vi "总磷氨氮测量数据储存.vi"   [LabVIEW 2016, in "斯坦道仪器.lvlib"]
types:
  T1 = cluster{"时间标识":timestamp, "监测值":sgl, "单位":u16, "数据标识":string, "因子编码":u32, "标样参考值":sgl, "F0":sgl, "F1":sgl, "F2":sgl, "F3":sgl, "F4":sgl, "F5":sgl, "F6":sgl, "F7":sgl, "X":sgl, "温度":sgl, "湿度":sgl, "量程标识":string}
  T2 = enum16{"维护数据", "水样测试", "标样核查", "零点核查", "跨度核查", "空白测试", "平行样测试", "加标回收", "空白校准", "标样校准", "初始化（清洗）"}
  T3 = cluster{"系统时间":timestamp, "工作状态":enum16{"空闲", "水样测试", "标样核查", "零点核查", "跨度核查", "空白测试", "平行样测试", "加标回收", "空白校准", "标样校准", "初始化（清洗）"}, "测量模式":enum16{"待机", "连续模式", "周期模式", "定点模式", "受控模式", "手动模式"}, "告警代码":enum16{"无告警", "缺试剂告警", "缺水样告警", "缺蒸馏水告警", "缺标液告警", "仪表漏液告警", "标定异常告警", "超量程告警", "加热异常", "低试剂预警", "超上限告警", "超下限告警", "仪表内部其他异常", "滴定异常告警", "电极异常告警", "量程切换告警", "参数设置告警", "PH电极电位异常", "电导率电极异常", "浊度光度异常", "溶解氧电极异常", "溶解氧光强异常", "温度异常告警", "PH异常告警", "溶解氧异常告警", "电导率异常告警", "浊度异常告警", "叶绿素异常告警", "藻密度异常告警", "蓝绿藻异常告警", "ORP异常告警", "氨氮异常告警", "清洁刷异常告警", "SD卡异常告警", "蓝牙异常告警", "Wifi异常告警", "流程异常告警"}, "故障代码":enum16{"无故障", "电机故障", "温度故障", "通讯故障", "滴定故障"}, "日志代码":u16, "软件版本":u16, "F0":sgl, "F1":sgl, "F2":sgl, "F3":sgl, "T":sgl, "H":sgl, "id":u16, "flowid":u16, "量程":u16}
  T4 = enum16{"空闲", "水样测试", "标样核查", "零点核查", "跨度核查", "空白测试", "平行样测试", "加标回收", "空白校准", "标样校准", "初始化（清洗）"}
  T5 = cluster{"因子编码":u32, "单位":u16, "标样参考值":sgl, "水样数据时间":timestamp, "水样实测值":sgl, "水样数据标识":string, "标样数据时间":timestamp, "标样实测值":sgl, "标样数据标识":string, "空白数据时间":timestamp, "空白实测值":sgl, "空白数据标识":string, "零点核查数据时间":timestamp, "零点核查实测值":sgl, "零点核查数据标识":string, "跨度核查数据时间":timestamp, "跨度核查实测值":sgl, "跨度核查数据标识":string, "加标回收数据时间":timestamp, "加标回收实测值":sgl, "加标回收数据标识":string, "平行样数据时间":timestamp, "平行样实测值":sgl, "平行样数据标识":string, "F0":sgl, "F1":sgl, "F2":sgl, "F3":sgl, "F4":sgl, "F5":sgl, "F6":sgl, "F7":sgl, "温度":sgl, "湿度":sgl, "X值":sgl}
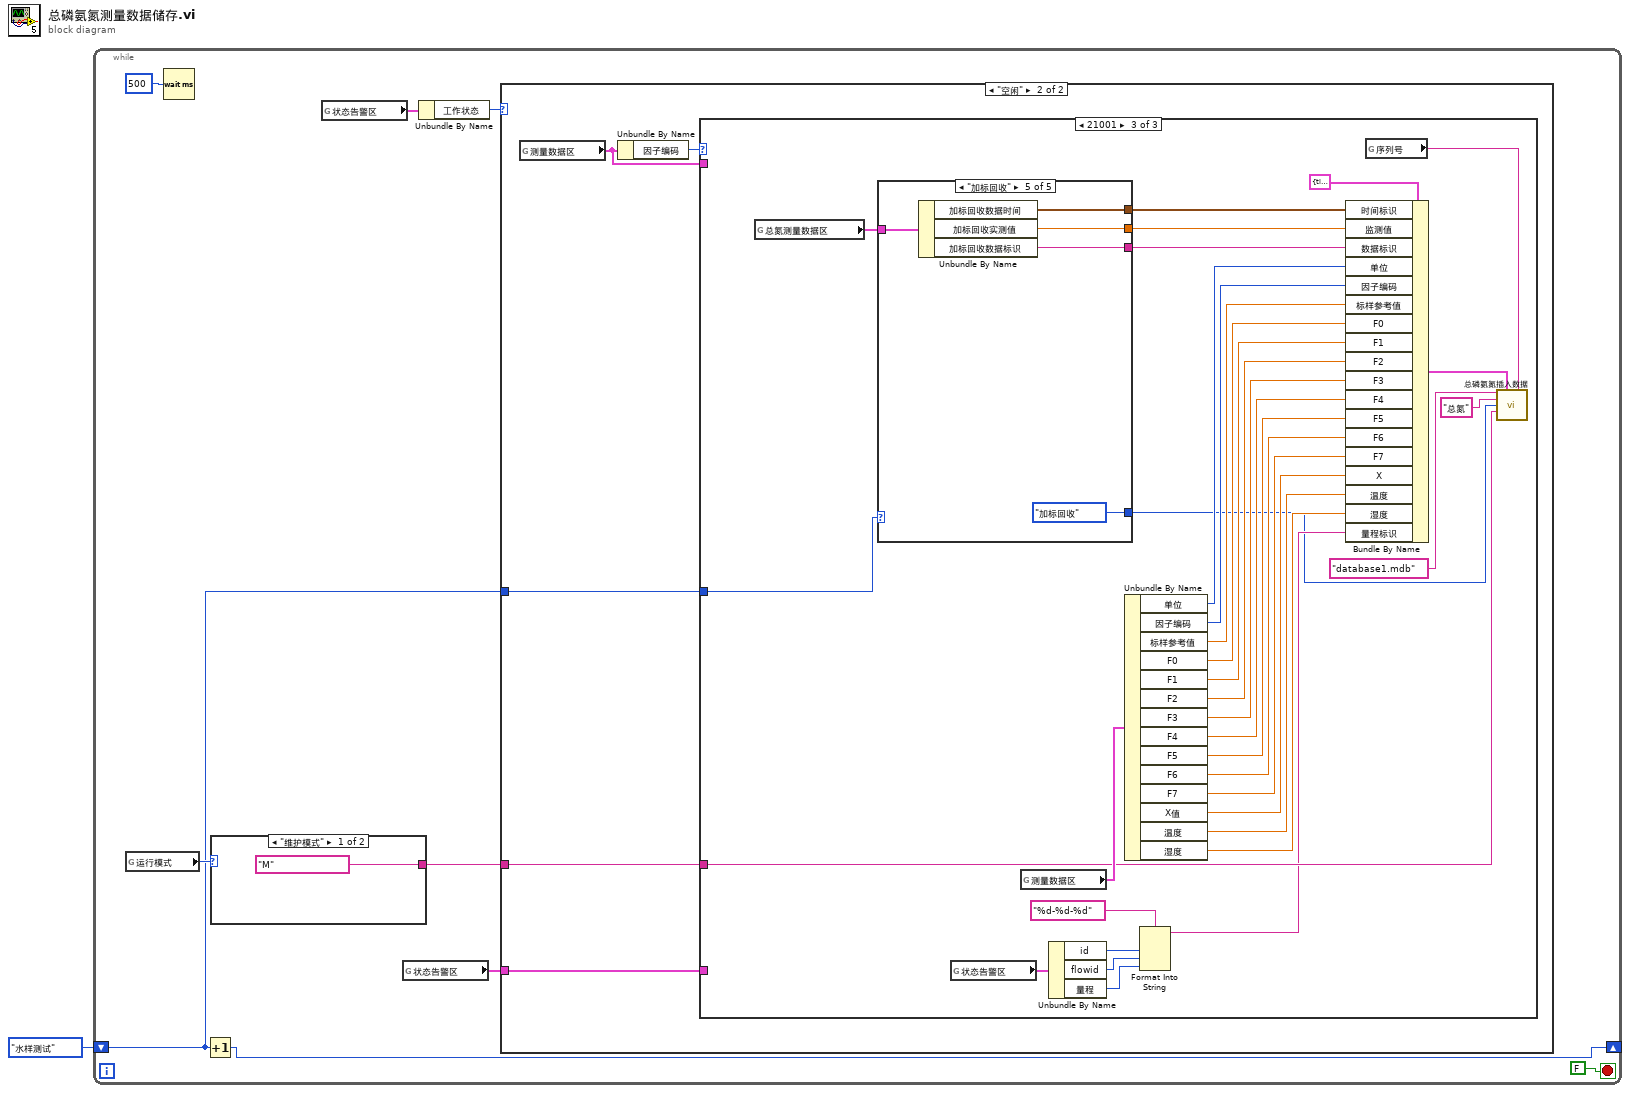
[diagram p0: block diagram]
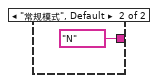
[diagram p2: hidden frame]
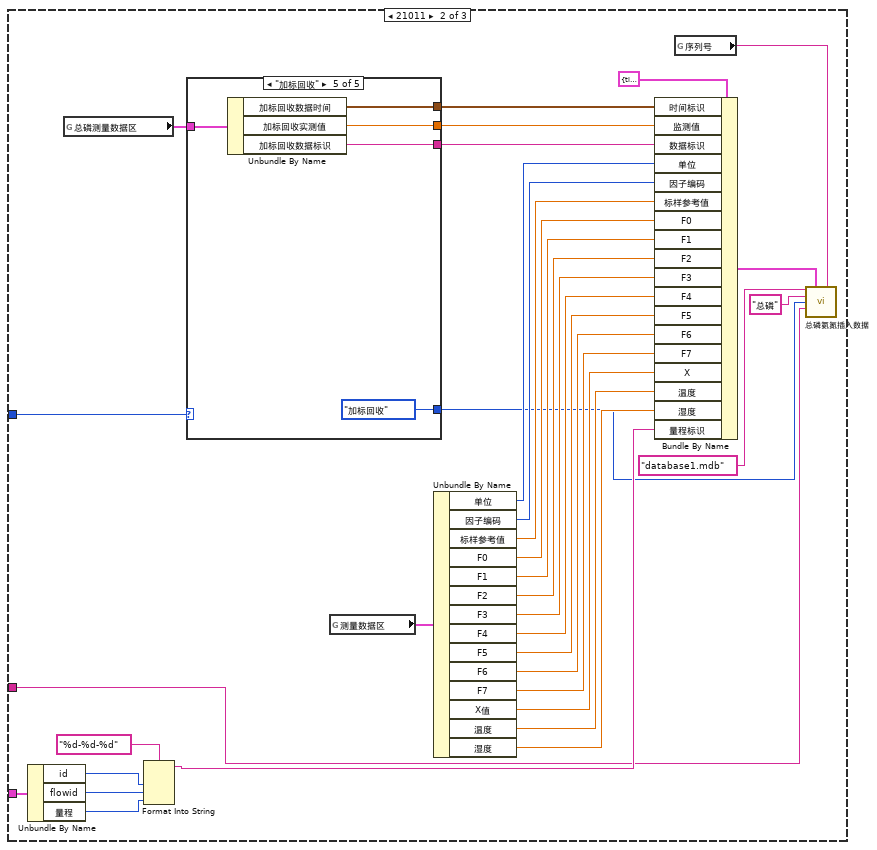
[diagram p5: hidden frame]
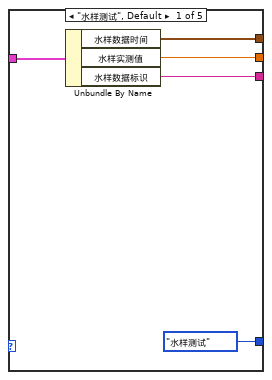
[diagram p6: hidden frame]
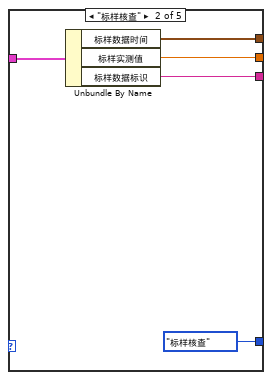
[diagram p7: hidden frame]
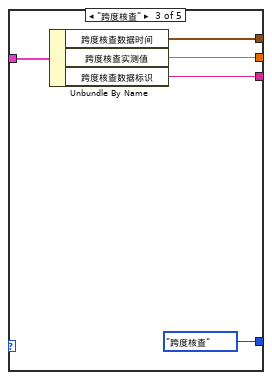
[diagram p8: hidden frame]
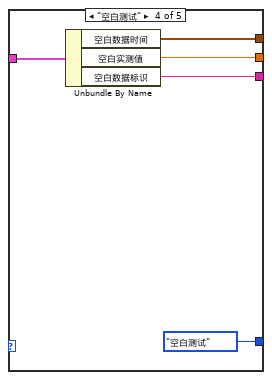
[diagram p9: hidden frame]
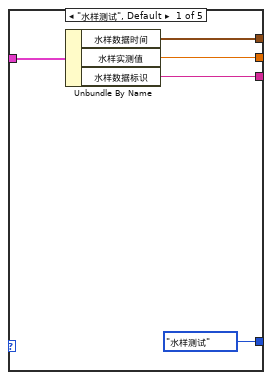
[diagram p10: hidden frame]
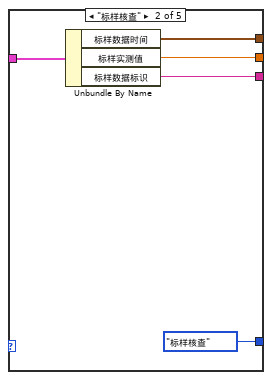
[diagram p11: hidden frame]
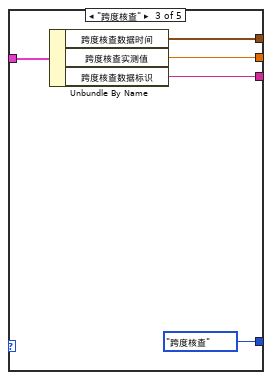
[diagram p12: hidden frame]
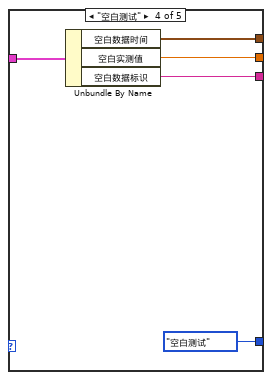
[diagram p13: hidden frame]
diagram:
  n1 = while {
    shift-right: [w4] -> _
    shift-left: enum16{"水样测试", "标样核查", "跨度核查", "空白测试", "加标回收"}."水样测试" ("测量模式") -> [w3]
    stop <- FALSE stop-if-true
    n2 = global read "系统变量.vi" "运行模式"() -> (w6:enum16{"维护模式", "常规模式", "应急模式", "质控模式"})
    n3 = Wait (ms)(milliseconds to wait=u32 500 ("等待时间（毫秒）")) -> ()  [unwired: 1 out]
    n4 = Increment(x=w3) -> (x+1=w4:enum16{"水样测试", "标样核查", "跨度核查", "空白测试", "加标回收"})
    n5 = case shown="\"维护模式\"" w6 {
      tunnel: ["M" ("数据标记表") "N" ("数据标记表")] -> w5
      frame "维护模式" {
      }
      frame "常规模式", Default {
      }
    }
    n6 = global read "VAR总磷氨氮全局变量.vi" "状态告警区"() -> (w8:T3)
    n7 = global read "VAR总磷氨氮全局变量.vi" "状态告警区"() -> (w2:T3)
    n8 = Unbundle By Name(w8) -> ("工作状态"=w7:T4)
    n9 = case shown="\"空闲\"" w7 {
      tunnel: w5 -> [_ w15]
      tunnel: w3 -> [_ w14]
      tunnel: w2 -> [_ w13]
      frame Default {
      }
      frame "空闲" {
        n10 = global read "VAR总磷氨氮全局变量.vi" "测量数据区"() -> (w17:T5)
        n11 = Unbundle By Name(w17) -> ("因子编码"=w16:u32)
        n12 = case shown="21001" w16 {
          tunnel: w17 -> [_ _ _]
          tunnel: w15 -> [_ w20 w96]
          tunnel: w14 -> [_ w19 w81]
          tunnel: w13 -> [_ w18 _]
          frame Default {
          }
          frame 21011 {
            n13 = Unbundle By Name(w18) -> ("id"=w50:u16, "flowid"=w33:u16, "量程"=w32:u16)
            n14 = global read "VAR总磷氨氮全局变量.vi" "总磷测量数据区"() -> (w49:T5)
            n15 = Format Into String(format string="%d-%d-%d" ("格式字符串"), w50, w33, w32) -> (resulting string=w34:string)  [unwired: 2 in, 1 out]
            n16 = case shown="\"加标回收\"" w19 {
              tunnel: w49 -> [w55 w60 w65 w70 w75]
              tunnel: [w54 w59 w64 w69 w74] -> w24
              tunnel: [w53 w58 w63 w68 w73] -> w25
              tunnel: [w52 w57 w62 w67 w72] -> w26
              tunnel: [T2."水样测试" ("测量模式") T2."标样核查" ("测量模式") T2."跨度核查" ("测量模式") T2."空白测试" ("测量模式") T2."加标回收" ("测量模式")] -> w23
              frame "水样测试", Default {
                n17 = Unbundle By Name(w55) -> ("水样数据时间"=w54:timestamp, "水样实测值"=w53:sgl, "水样数据标识"=w52:string)
              }
              frame "标样核查" {
                n18 = Unbundle By Name(w60) -> ("标样数据时间"=w59:timestamp, "标样实测值"=w58:sgl, "标样数据标识"=w57:string)
              }
              frame "跨度核查" {
                n19 = Unbundle By Name(w65) -> ("跨度核查数据时间"=w64:timestamp, "跨度核查实测值"=w63:sgl, "跨度核查数据标识"=w62:string)
              }
              frame "空白测试" {
                n20 = Unbundle By Name(w70) -> ("空白数据时间"=w69:timestamp, "空白实测值"=w68:sgl, "空白数据标识"=w67:string)
              }
              frame "加标回收" {
                n21 = Unbundle By Name(w75) -> ("加标回收数据时间"=w74:timestamp, "加标回收实测值"=w73:sgl, "加标回收数据标识"=w72:string)
              }
            }
            n22 = global read "VAR总磷氨氮全局变量.vi" "测量数据区"() -> (w31:T5)
            n23 = Unbundle By Name(w31) -> ("单位"=w48:u16, "因子编码"=w47:u32, "标样参考值"=w46:sgl, "F0"=w45:sgl, "F1"=w44:sgl, "F2"=w43:sgl, "F3"=w42:sgl, "F4"=w41:sgl, "F5"=w40:sgl, "F6"=w39:sgl, "F7"=w38:sgl, "X值"=w37:sgl, "温度"=w36:sgl, "湿度"=w35:sgl)
            n24 = Bundle By Name(cluster=T1 {"时间标识"=timestamp(0 s since 1904-01-01), "监测值"=0.0, "单位"=0, "数据标识"="", "因子编码"=0, "标样参考值"=0.0, "F0"=0.0, "F1"=0.0, "F2"=0.0, "F3"=0.0, "F4"=0.0, "F5"=0.0, "F6"=0.0, "F7"=0.0, "X"=0.0, "温度"=0.0, "湿度"=0.0, "量程标识"=""} ("data"), "时间标识"=w24, "监测值"=w25, "数据标识"=w26, "单位"=w48, "因子编码"=w47, "标样参考值"=w46, "F0"=w45, "F1"=w44, "F2"=w43, "F3"=w42, "F4"=w41, "F5"=w40, "F6"=w39, "F7"=w38, "X"=w37, "温度"=w36, "湿度"=w35, "量程标识"=w34) -> (w28:T1)
            n25 = global read "VAR总磷氨氮全局变量.vi" "序列号"() -> (w27:string)
            n26 = call "总磷氨氮插入数据.vi"("database"="database1.mdb", "data"=w28, "SN"=w27, "table"="总磷", "测量模式"=w23, "数据标记表"=w20) -> ()  [unwired: 9 in, 1 out]
          }
          frame 21001 {
            n27 = global read "VAR总磷氨氮全局变量.vi" "总氮测量数据区"() -> (w80:T5)
            n28 = case shown="\"加标回收\"" w81 {
              tunnel: w80 -> [w113 w118 w123 w128 w133]
              tunnel: [w112 w117 w122 w127 w132] -> w79
              tunnel: [w111 w116 w121 w126 w131] -> w78
              tunnel: [w110 w115 w120 w125 w130] -> w77
              tunnel: [T2."水样测试" ("测量模式") T2."标样核查" ("测量模式") T2."跨度核查" ("测量模式") T2."空白测试" ("测量模式") T2."加标回收" ("测量模式")] -> w76
              frame "水样测试", Default {
                n29 = Unbundle By Name(w113) -> ("水样数据时间"=w112:timestamp, "水样实测值"=w111:sgl, "水样数据标识"=w110:string)
              }
              frame "标样核查" {
                n30 = Unbundle By Name(w118) -> ("标样数据时间"=w117:timestamp, "标样实测值"=w116:sgl, "标样数据标识"=w115:string)
              }
              frame "跨度核查" {
                n31 = Unbundle By Name(w123) -> ("跨度核查数据时间"=w122:timestamp, "跨度核查实测值"=w121:sgl, "跨度核查数据标识"=w120:string)
              }
              frame "空白测试" {
                n32 = Unbundle By Name(w128) -> ("空白数据时间"=w127:timestamp, "空白实测值"=w126:sgl, "空白数据标识"=w125:string)
              }
              frame "加标回收" {
                n33 = Unbundle By Name(w133) -> ("加标回收数据时间"=w132:timestamp, "加标回收实测值"=w131:sgl, "加标回收数据标识"=w130:string)
              }
            }
            n34 = global read "VAR总磷氨氮全局变量.vi" "状态告警区"() -> (w104:T3)
            n35 = global read "VAR总磷氨氮全局变量.vi" "测量数据区"() -> (w108:T5)
            n36 = Unbundle By Name(w104) -> ("id"=w100:u16, "flowid"=w99:u16, "量程"=w98:u16)
            n37 = Unbundle By Name(w108) -> ("单位"=w107:u16, "因子编码"=w106:u32, "标样参考值"=w105:sgl, "F0"=w94:sgl, "F1"=w93:sgl, "F2"=w92:sgl, "F3"=w91:sgl, "F4"=w90:sgl, "F5"=w89:sgl, "F6"=w88:sgl, "F7"=w87:sgl, "X值"=w86:sgl, "温度"=w85:sgl, "湿度"=w84:sgl)
            n38 = Format Into String(format string="%d-%d-%d" ("格式字符串"), w100, w99, w98) -> (resulting string=w83:string)  [unwired: 2 in, 1 out]
            n39 = Bundle By Name(cluster=T1 {"时间标识"=timestamp(0 s since 1904-01-01), "监测值"=0.0, "单位"=0, "数据标识"="", "因子编码"=0, "标样参考值"=0.0, "F0"=0.0, "F1"=0.0, "F2"=0.0, "F3"=0.0, "F4"=0.0, "F5"=0.0, "F6"=0.0, "F7"=0.0, "X"=0.0, "温度"=0.0, "湿度"=0.0, "量程标识"=""} ("data"), "时间标识"=w79, "监测值"=w78, "数据标识"=w77, "单位"=w107, "因子编码"=w106, "标样参考值"=w105, "F0"=w94, "F1"=w93, "F2"=w92, "F3"=w91, "F4"=w90, "F5"=w89, "F6"=w88, "F7"=w87, "X"=w86, "温度"=w85, "湿度"=w84, "量程标识"=w83) -> (w82:T1)
            n40 = global read "VAR总磷氨氮全局变量.vi" "序列号"() -> (w97:string)
            n41 = call "总磷氨氮插入数据.vi"("database"="database1.mdb", "data"=w82, "SN"=w97, "table"="总氮", "测量模式"=w76, "数据标记表"=w96) -> ()  [unwired: 9 in, 1 out]
          }
        }
      }
    }
  }
